vi "XNET Bus Monitor Server.vi"() -> ()   [LabVIEW 2025]
uses:
  <resource>/objmgr/xnet.rc
  Support Code/XNET.CAN.BusMonitor.API.lvlib
panel:
  out "error out":errorcluster
  out "Instances":i32
  in  "Stop":bool
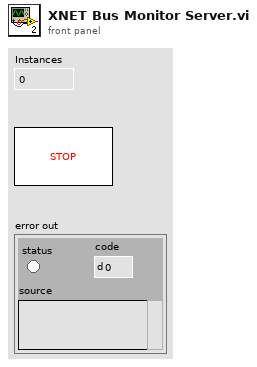
[diagram p1: front panel]
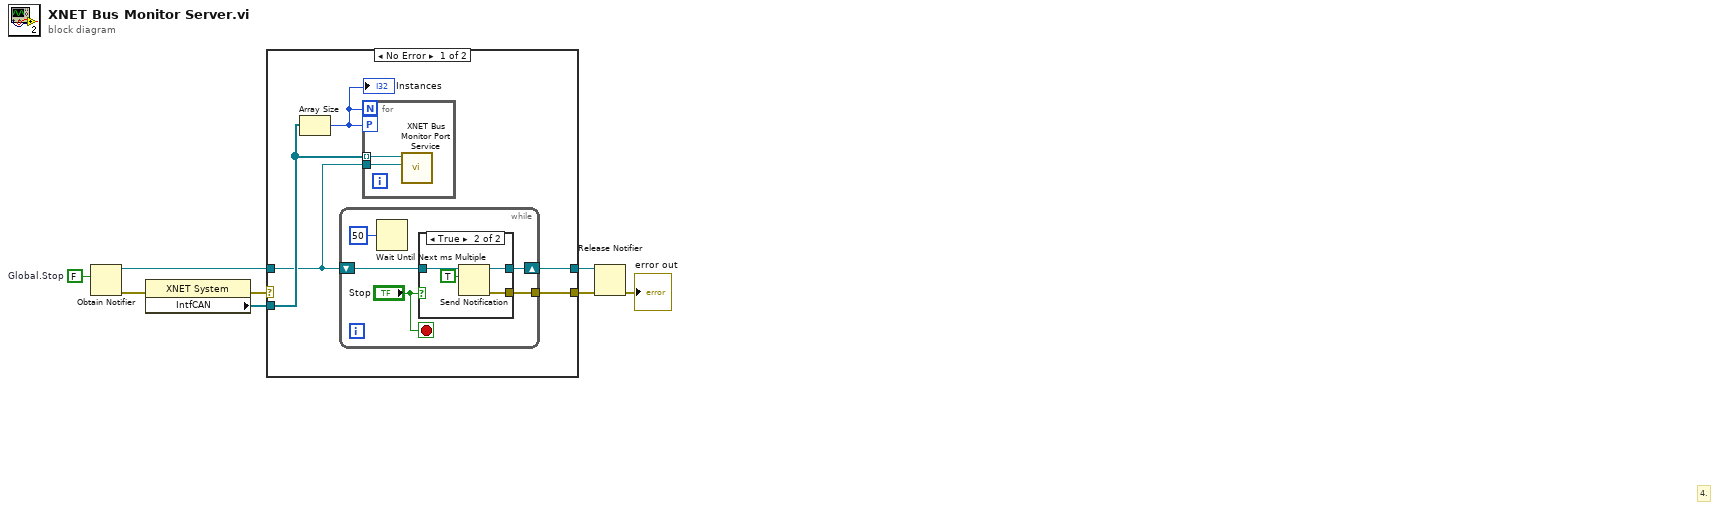
[diagram p0: block diagram]
diagram:
  w7 = FALSE  # Global.Stop
  # "4."
  n1 = Obtain Notifier(notification data type=w7) -> (notifier out=w5:refnum<notifier>, error out=w6:errorcluster)  [unwired: 3 in, 1 out]
  n2 = property class="XNET System"(error in=w6) -> (error out=w4:errorcluster, "IntfCAN"=w8:refnum<k21>[])  [unwired: 1 in, 1 out]
  n3 = case shown="No Error" w4 {
    selector: w4 -> [_ w26]
    tunnel: w8 -> [w13 _]
    tunnel: w5 -> [w11 w27]
    tunnel: [w10 w27] -> w3
    tunnel: [w9 w26] -> w2
    frame No Error {
      n4 = Array Size(array=w13) -> (size(s)=w12:i32)
      "Instances" <- w12
      n5 = while {
        shift-right: [w15] -> w10
        shift-left: w11 -> [w18]
        tunnel: [w14] -> w9
        stop <- "Stop" stop-if-true
        n6 = Wait Until Next ms Multiple(millisecond multiple=u32 50) -> ()  [unwired: 1 out]
        n7 = case shown="True" "Stop" {
          tunnel: w18 -> [w19 w23]
          tunnel: [w19 w22] -> w15
          tunnel: [_ w21] -> w14
          frame False {
          }
          frame True {
            n8 = Send Notification(notification=TRUE, notifier=w23) -> (notifier out=w22:refnum<notifier>, error out=w21:errorcluster)  [unwired: 1 in]
          }
        }
      }
      n9 = for {
        N: w12 -> [_]
        tunnel: w13 -> [w25] mode=indexing
        workers-P: w12 -> [_]
        tunnel: w11 -> [w24]
        n10 = call "XNET Bus Monitor Port Service.vi"("Global Stop"=w24, "Name in"=w25) -> ()  [unwired: 10 in]
      }
    }
    frame Error {
    }
  }
  n11 = Release Notifier(notifier=w3, error in (no error)=w2) -> (error out=→"error out":errorcluster)  [unwired: 1 in, 2 out]
